vi "publish -- stepper position -- eventful.vi"(0 "step (fdeg)":dbl=1000.0 format="%#_10f", 1 "publisher action":T1) -> (4 "step out (Hz)":dbl=1000.0 format="%#_10f", 10 "response event":refnum<user-event>, 14 "response type":cluster{"step (fdeg)":dbl}={"step (fdeg)"=1000.0}, 15 "request event":refnum<user-event>)   [LabVIEW 2020]
uses:
  publisher action.ctl
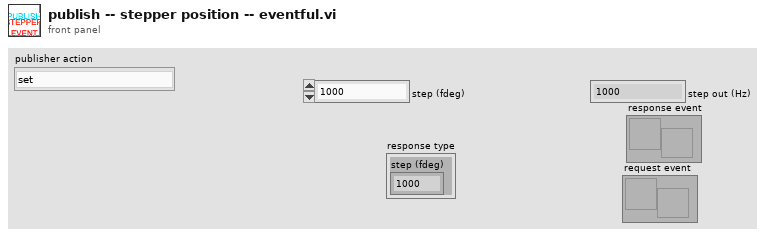
[diagram p1: front panel]
types:
  T1 = typedef "publisher action.ctl" = enum16{"set", "get", "init", "check"}
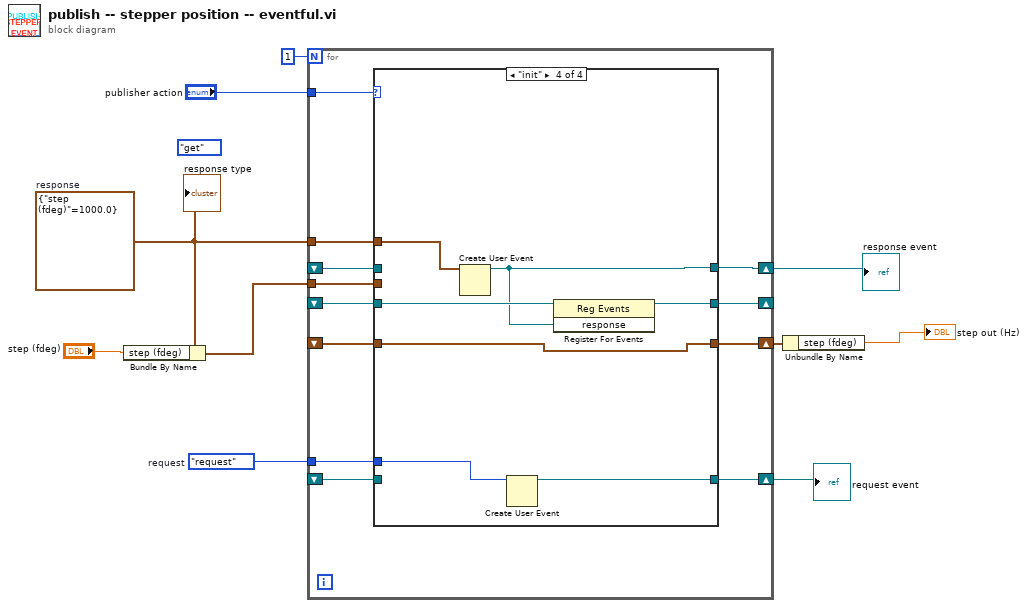
[diagram p0: block diagram]
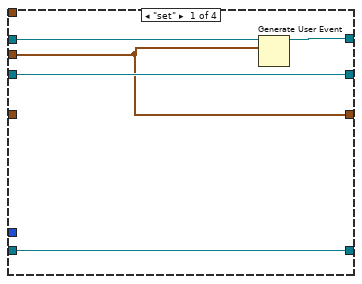
[diagram p2: hidden frame]
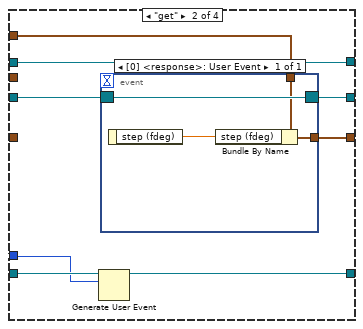
[diagram p3: hidden frame]
diagram:
  w5 = cluster{"step (fdeg)":dbl} {"step (fdeg)"=1000.0}  # response
  w8 = enum16{"request"}."request"  # request
  (unwired) publisher_action."get" ("publisher action")
  n1 = Bundle By Name(cluster=w5, "step (fdeg)"="step (fdeg)") -> (w3:cluster{"step (fdeg)":dbl})
  n2 = for {
    N: 1 -> [_]
    tunnel: "publisher action" -> [w22]
    tunnel: w3 -> [w21]
    shift-right: [w12] -> w2
    shift-left: _ -> [w20]
    shift-right: [w11] -> w6
    shift-left: _ -> [w13]
    shift-right: [w14] -> w7
    shift-left: _ -> [w19]
    shift-right: [w18] -> _
    shift-left: _ -> [w17]
    tunnel: w8 -> [w16]
    tunnel: w5 -> [w15]
    n3 = case shown="\"init\"" w22 {
      tunnel: w21 -> [w24 _ _ _]
      tunnel: w20 -> [_ _ w41 w46]
      tunnel: w13 -> [w25 w28 w40 _]
      tunnel: w19 -> [w26 w33 w42 _]
      tunnel: [w27 w35 w43 w47] -> w18
      tunnel: w17 -> [w27 w34 w43 w45]
      tunnel: w16 -> [_ w32 _ w49]
      tunnel: w15 -> [_ w30 _ w50]
      tunnel: [w26 w31 w42 w48] -> w14
      tunnel: [w24 w29 w41 w46] -> w12
      tunnel: [w23 w28 w40 w44] -> w11
      frame "set" {
        n4 = Generate User Event(user event=w25, event data cluster=w24) -> (user event out=w23:refnum<user-event>)  [unwired: 2 in, 1 out]
      }
      frame "get" {
        n5 = Generate User Event(user event=w33, event data cluster=w32) -> (user event out=w31:refnum<user-event>)  [unwired: 2 in, 1 out]
        n6 = event shown="[0] <response>: User Event" {
          selector: w34 -> [w39]
          dyn-events: [w39] -> w35
          timeout: _ -> [_]
          tunnel: w30 -> [w37]
          tunnel: [w36] -> w29
          event User Event {
            n7 = event-data() -> ("step (fdeg)"=w38:dbl)  [unwired: 1 in]
            n8 = Bundle By Name(cluster=w37, "step (fdeg)"=w38) -> (w36:cluster{"step (fdeg)":dbl})
          }
        }
      }
      frame "check", Default {
      }
      frame "init" {
        n9 = Create User Event(user event datatype=w50) -> (user event=w44:refnum<user-event>)  [unwired: 1 in, 1 out]
        n10 = Create User Event(user event datatype=w49) -> (user event=w48:refnum<user-event>)  [unwired: 1 in, 1 out]
        n11 = register-events(reference=w45, w44) -> (reference out=w47:refnum<event-registration>)  [unwired: 1 in, 1 out]
      }
    }
  }
  "request event" <- w7
  "response event" <- w6
  n12 = Unbundle By Name(w2) -> ("step (fdeg)"=→"step out (Hz)":dbl)
  "response type" <- w5
